vi "XYZStage-Initialisation.vi"(8 "Error In":errorcluster, 10 "Z Stage":T2, 11 "XY Stage":T3) -> (0 "Error Out":errorcluster, 3 "VISA resource name out XY":refnum<visa-resource-name>)   [LabVIEW 2020]
uses:
  Typedefs/XY Stage config cluster.ctl
  Typedefs/Z Stage config cluster.ctl
  Typedefs/Comms settings-rs232.ctl
  Global Variables/General Globals.vi
  <vilib>/Instr/_visa.llb/VISA Configure Serial Port (Instr).vi
  Globals/gl_XYZStage globals.vi
  Drivers/Olympus IX BX Series/Olympus IX BX Series.lvlib
panel:
  in  "Connection Z":T1={"baud rate"=9600, "data bits"=8, "parity"=0, "stop bits"=10, "flow control"=0} {"flow control" items=["None"=0, "XON/XOFF"=1, "RTS/CTS"=2, "DTR/DSR"=4]; "stop bits" items=["1.0"=10, "1.5"=15, "2.0"=20]; "parity" items=["None", "Odd", "Even", "Mark", "Space"]; "data bits" min=5 max=8 step=1}
  out "VISA resource name out Z":refnum<visa-resource-name>
  in  "Connection Z":T1={"baud rate"=9600, "data bits"=8, "parity"=0, "stop bits"=10, "flow control"=0} {"flow control" items=["None"=0, "XON/XOFF"=1, "RTS/CTS"=2, "DTR/DSR"=4]; "stop bits" items=["1.0"=10, "1.5"=15, "2.0"=20]; "parity" items=["None", "Odd", "Even", "Mark", "Space"]; "data bits" min=5 max=8 step=1}
  in  "Connection XY":T1={"baud rate"=9600, "data bits"=8, "parity"=0, "stop bits"=10, "flow control"=0} {"flow control" items=["None"=0, "XON/XOFF"=1, "RTS/CTS"=2, "DTR/DSR"=4]; "stop bits" items=["1.0"=10, "1.5"=15, "2.0"=20]; "parity" items=["None", "Odd", "Even", "Mark", "Space"]; "data bits" min=5 max=8 step=1}
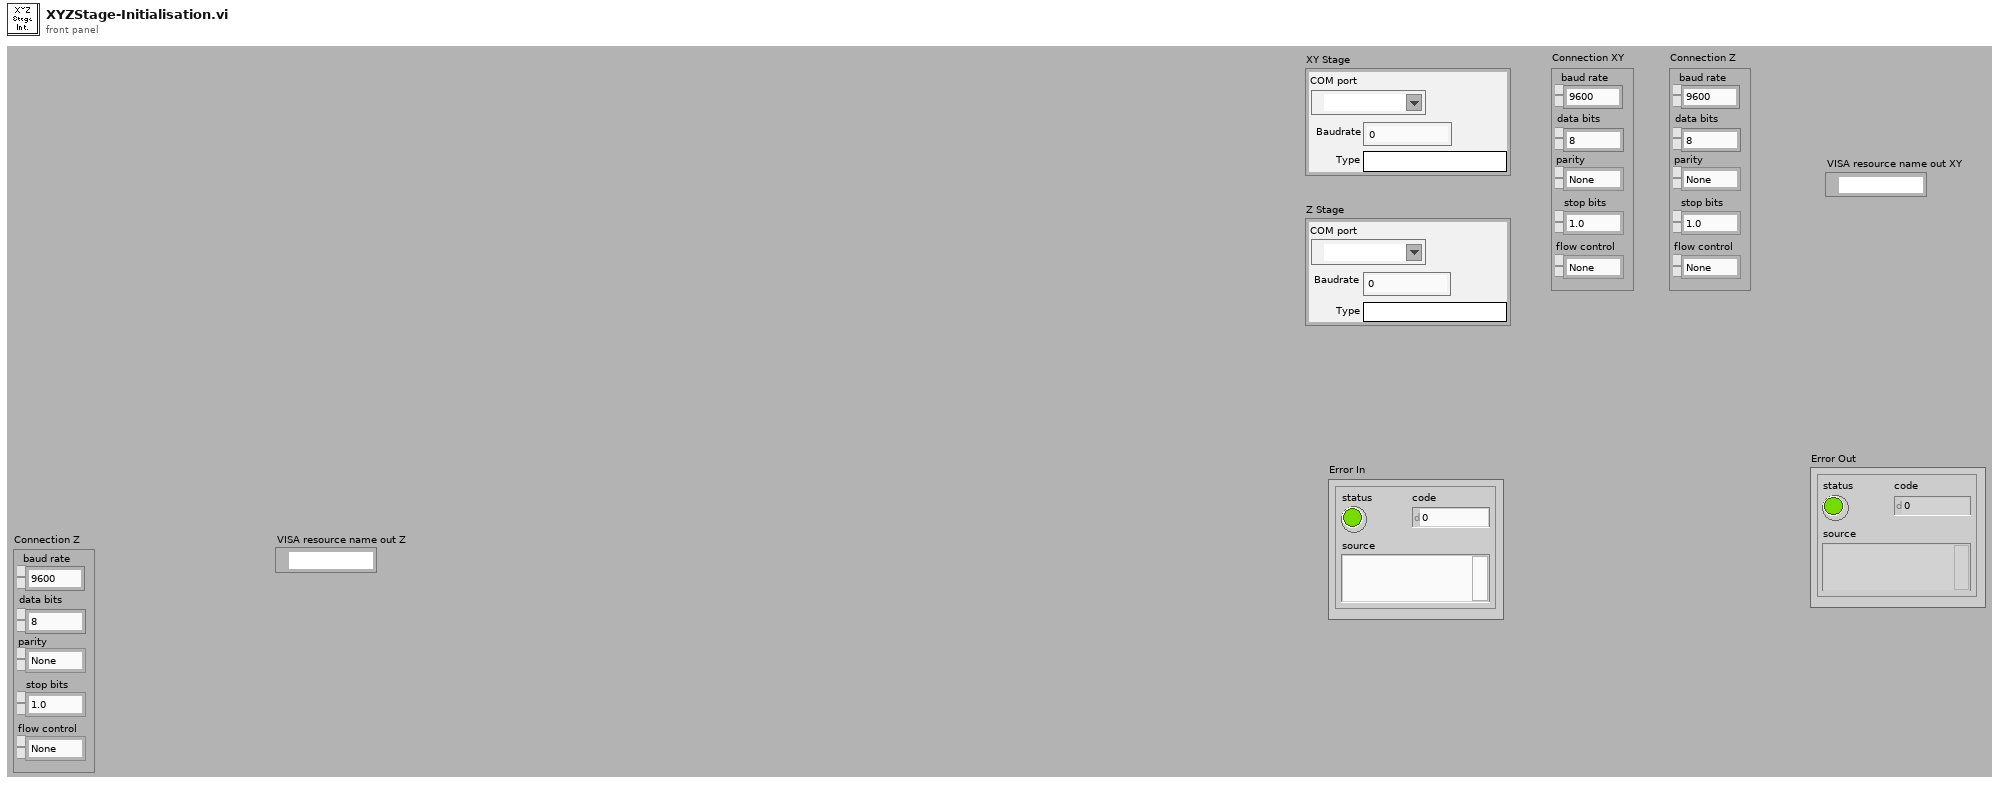
[diagram p1: front panel]
types:
  T1 = typedef "Comms settings-rs232.ctl" = cluster{"baud rate":u32, "data bits":u16, "parity":u16, "stop bits":u16, "flow control":u16}
  T2 = typedef "Z Stage config cluster.ctl" = cluster{"COM port":refnum<visa-resource-name>, "Baudrate":i32, "Type":string}
  T3 = typedef "XY Stage config cluster.ctl" = cluster{"COM port":refnum<visa-resource-name>, "Baudrate":i32, "Type":string}
  T4 = cluster{"Baud Rate (19200)":u32, "Flow Control (2: RTS/CTS)":u16, "Parity (2: Even)":u16, "Data Bits (8)":u16, "Stop Bits (20: 2.0)":u16}
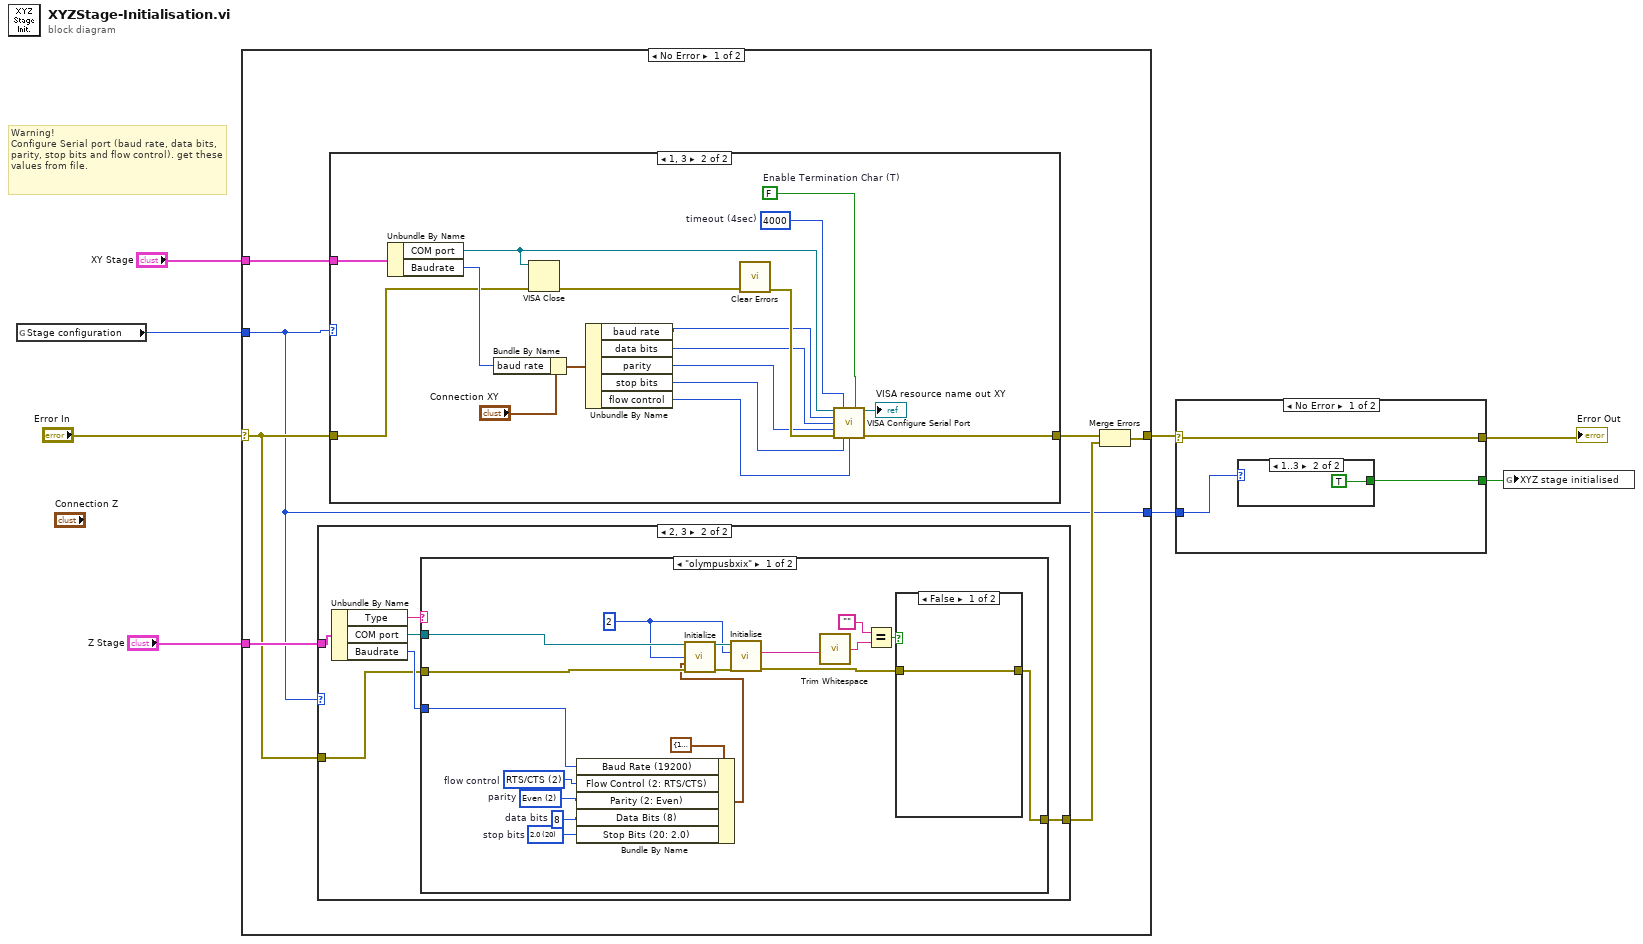
[diagram p0: block diagram]
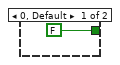
[diagram p2: hidden frame]
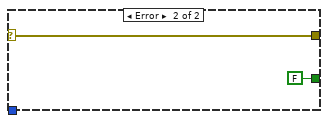
[diagram p3: hidden frame]
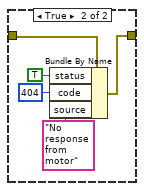
[diagram p5: hidden frame]
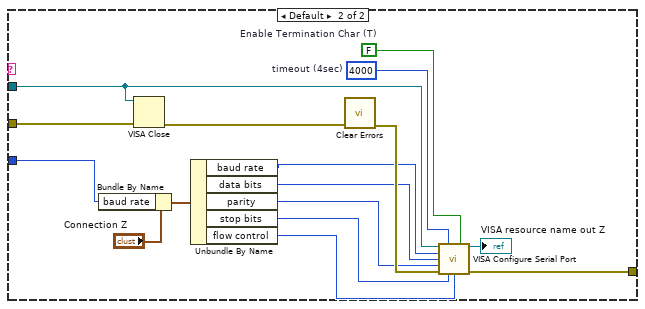
[diagram p6: hidden frame]
diagram:
  # "Warning!\nConfigure Serial port (baud rate, data bits, parity, stop bits and flow control). get these values from file."
  n1 = global read "General Globals.vi" "Stage configuration"() -> (w6:i32)
  n2 = case shown="No Error" "Error In" {
    selector: "Error In" -> [w13 w82]
    tunnel: [w10 w82] -> w4
    tunnel: "XY Stage" -> [w15 _]
    tunnel: w6 -> [w9 w81]
    tunnel: "Z Stage" -> [w14 _]
    tunnel: [w9 w81] -> w3
    frame No Error {
      n3 = case shown="2, 3" w9 {
        tunnel: w14 -> [_ w20]
        tunnel: w13 -> [w16 w19]
        tunnel: [w16 w18] -> w11
        frame 0, Default {
        }
        frame 2, 3 {
          n4 = Unbundle By Name(w20) -> ("Type"=w17:string, "COM port"=w22:refnum<visa-resource-name>, "Baudrate"=w21:i32)
          n5 = case shown="\"olympusbxix\"" w17 {
            tunnel: w22 -> [w35 w59]
            tunnel: w21 -> [w36 w55]
            tunnel: w19 -> [w38 w50]
            tunnel: [w30 w49] -> w18
            frame "olympusbxix" {
              w28 = u16 8  # data bits
              w27 = u16 2 items=["None", "Odd", "Even", "Mark", "Space"]  # parity
              w26 = u16 20 items=["1.0"=10, "1.5"=15, "2.0"=20]  # stop bits
              w25 = u16 2 items=["None"=0, "XON/XOFF"=1, "RTS/CTS"=2, "DTR/DSR"=4]  # flow control
              w29 = 2 ("Device Number (1)")
              n6 = Bundle By Name(cluster=T4 {"Baud Rate (19200)"=19200, "Flow Control (2: RTS/CTS)"=2, "Parity (2: Even)"=2, "Data Bits (8)"=8, "Stop Bits (20: 2.0)"=20} ("Serial Configuration"), "Baud Rate (19200)"=w36, "Flow Control (2: RTS/CTS)"=w25, "Parity (2: Even)"=w27, "Data Bits (8)"=w28, "Stop Bits (20: 2.0)"=w26) -> (w34:T4)
              n7 = call "Initialize.vi"("VISA Resource Name"=w35, "Device Number (1)"=w29, "Serial Configuration"=w34, "error in (no error)"=w38) -> ("VISA Resource Name Out"=w40:refnum<visa-resource-name>, "error out"=w39:errorcluster)  [unwired: 10 in]
              n8 = call "Initialise.vi"("error in (no error)"=w39, "Device Number (1)"=w29, "VISA Resource Name"=w40) -> ("error out"=w24:errorcluster, "Result"=w23:string)  [unwired: 6 in, 1 out]
              n9 = call <vilib>:"Trim Whitespace.vi"("string"=w23) -> ("trimmed string"=w33:string)  [unwired: 1 in]
              n10 = Equal?(x="", y=w33) -> (x = y?=w31:bool)
              n11 = case shown="False" w31 {
                tunnel: w24 -> [w41 w46]
                tunnel: [w41 w45] -> w30
                frame False {
                }
                frame True {
                  n12 = Bundle By Name(cluster=w46, "status"=TRUE, "code"=404, "source"="No response from motor") -> (w45:errorcluster)
                }
              }
            }
            frame Default {
              w60 = FALSE  # Enable Termination Char (T)
              w61 = u32 4000  # timeout (4sec)
              n13 = Bundle By Name(cluster="Connection Z", "baud rate"=w55) -> (w54:T1)
              n14 = VISA Close(VISA resource name=w59, error in (no error)=w50) -> (error out=w58:errorcluster)
              n15 = Unbundle By Name(w54) -> ("baud rate"=w53:u32, "data bits"=w52:u16, "parity"=w51:u16, "stop bits"=w48:u16, "flow control"=w47:u16)
              n16 = call <vilib>:"Clear Errors.vi"("error in (no error)"=w58) -> ("error out"=w57:errorcluster)  [unwired: 5 in, 1 out]
              n17 = call-poly "VISA Configure Serial Port"("VISA resource name"=w59, "timeout (10sec)"=w61, "Enable Termination\nChar (T)"=w60, "baud rate (9600)"=w53, "data bits (8)"=w52, "parity (0:none)"=w51, "error in (no error)"=w57, "stop bits (10: 1 bit)"=w48, "flow control (0:none)"=w47) -> ("VISA resource name out"=→"VISA resource name out Z":refnum<visa-resource-name>, "error out"=w49:errorcluster)  [unwired: 5 out]
            }
          }
        }
      }
      n18 = case shown="1, 3" w9 {
        tunnel: [w63 w77] -> w12
        tunnel: w15 -> [_ w76]
        tunnel: w13 -> [w63 w66]
        frame 0, Default {
        }
        frame 1, 3 {
          w78 = FALSE  # Enable Termination Char (T)
          w79 = u32 4000  # timeout (4sec)
          n19 = Unbundle By Name(w76) -> ("COM port"=w75:refnum<visa-resource-name>, "Baudrate"=w71:i32)
          n20 = Bundle By Name(cluster="Connection XY", "baud rate"=w71) -> (w70:T1)
          n21 = VISA Close(VISA resource name=w75, error in (no error)=w66) -> (error out=w74:errorcluster)
          n22 = Unbundle By Name(w70) -> ("baud rate"=w69:u32, "data bits"=w68:u16, "parity"=w67:u16, "stop bits"=w65:u16, "flow control"=w64:u16)
          n23 = call <vilib>:"Clear Errors.vi"("error in (no error)"=w74) -> ("error out"=w73:errorcluster)  [unwired: 5 in, 1 out]
          n24 = call-poly "VISA Configure Serial Port"("VISA resource name"=w75, "timeout (10sec)"=w79, "Enable Termination\nChar (T)"=w78, "baud rate (9600)"=w69, "data bits (8)"=w68, "parity (0:none)"=w67, "error in (no error)"=w73, "stop bits (10: 1 bit)"=w65, "flow control (0:none)"=w64) -> ("VISA resource name out"=→"VISA resource name out XY":refnum<visa-resource-name>, "error out"=w77:errorcluster)  [unwired: 5 out]
        }
      }
      n25 = Merge Errors(w12, w11) -> (w10:errorcluster)
    }
    frame Error {
    }
  }
  n26 = case shown="No Error" w4 {
    selector: w4 -> [w83 w88]
    tunnel: w3 -> [w85 _]
    tunnel: [w84 FALSE ("XYZ stage initialised")] -> w2
    tunnel: [w83 w88] -> w1
    frame No Error {
      n27 = case shown="1..3" w85 {
        tunnel: [FALSE TRUE ("XYZ stage initialised")] -> w84
        frame 0, Default {
        }
        frame 1..3 {
        }
      }
    }
    frame Error {
    }
  }
  "Error Out" <- w1
  n28 = global write "gl_XYZStage globals.vi" "XYZ stage initialised"(w2) -> ()
